vi "PCSLauncher.constructor.vi"(0 "name":string, 2 "data in":string, 5 "error in(no error)":errorcluster) -> (14 "i ref out":refnum<vi>, 16 "data out":string, 19 "error out":errorcluster)   [LabVIEW 2014, in "PCSLauncher.lvlib"]
doc: "This class is forseen to control black boxes (motion).\n\nThis class is part of the PHELIX device layer.\n\nauthor: Stefan Götte, GSI\n\nLicense Agreement for this software:\n\nCopyright (C)\nGesellschaft für Schwerionenforschung, GSI\nPlanckstr. 1\n64291 Darmstadt\nGermany\n\nContact: D.Beck@gsi.de \n\nThis program is free software; you can redistribute it and/or modify it under the terms of the \nGNU General Public License as published by the Free Software Foundation; either version 2 of \nthe license, or (at your option) any later version.\n\nThis program is distributed in the hope that it will be useful, but WITHOUT ANY WARRANTY; \nwithout even the implied warranty of MERCHANTABILITY or FITNESS FOR A PARTICULAR PURPOSE. See the GNU General License for more details (http://www.gnu.org).\n\nGesellschaft für Schwerionenforschung, GSI\nPlanckstr. 1, 64291 Darmstadt, Germany\nFor all questions and ideas contact: M.Richter@gsi.de, H.Brand@gsi.de or D.Beck@gsi.de.\nLast update: 16-JUN-2004"
uses:
  PCSLauncher.lvlib
  CSCore/CSObj/CSObj.lvlib
  PH_Class/PH_Class.lvlib
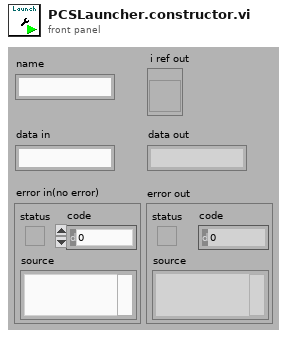
[diagram p1: front panel]
types:
  T1 = enum16{"SetAttribute", "GetAttribute", "CreateAttribute", "DestroyAttribute", "DestroyAllAtributes"}
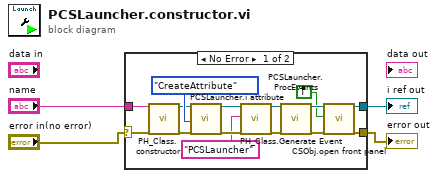
[diagram p0: block diagram]
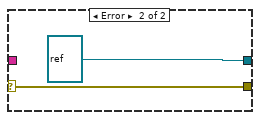
[diagram p2: hidden frame]
diagram:
  n1 = case shown="No Error" "error in(no error)" {
    selector: "error in(no error)" -> [w16 w21]
    tunnel: [w9 refnum<vi> refnum ("i ref out")] -> w4
    tunnel: [w11 w21] -> w3
    tunnel: "name" -> [w15 _]
    frame No Error {
      n2 = call "PH_Class.constructor.vi"("name"=w15, "error in"=w16) -> ("i ref out"=w17:refnum<vi>, "error out"=w18:errorcluster)  [unwired: 15 in, 1 out]
      n3 = call "PCSLauncher.i attribute.vi"("VI Refnum"=w17, "Action"=T1."CreateAttribute", "error in (no error)"=w18) -> ("VI Refnum out"=w5:refnum<vi>, "error out"=w7:errorcluster)  [unwired: 14 in, 1 out]
      n4 = call "PH_Class.Generate Event.vi"("i ref in"=w5, "Class"="PCSLauncher", "error in (no error)"=w7) -> ("i ref out"=w14:refnum<vi>, "error out"=w13:errorcluster)  [unwired: 15 in]
      n5 = call "PCSLauncher.ProcEvents.vi"("i ref in"=w14, "error in (no error)"=w13) -> ("i ref out"=w10:refnum<vi>, "error out"=w12:errorcluster)  [unwired: 16 in]
      n6 = call "CSObj.open front panel.vi"("i ref in"=w10, "frontPanelOpen"=TRUE, "error in (no error)"=w12) -> ("i ref out"=w9:refnum<vi>, "error out"=w11:errorcluster)  [unwired: 15 in]
    }
    frame Error {
    }
  }
  "i ref out" <- w4
  "error out" <- w3
